vi "Stop Arrival Time TIO.vi"(8 "error in":errorcluster, 10 "Temp File Definition":T1, 11 "Arrival Time Clusters":T2(array[cluster])) -> (0 "error out":errorcluster, 3 "Temp File Definition Out":T1)   [LabVIEW 2009]
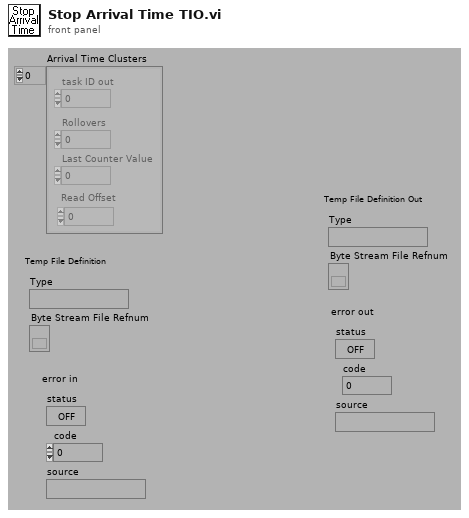
[diagram p1: front panel]
types:
  T1 = cluster{"Type":string, "Byte Stream File Refnum":refnum<file>}
  T2 = cluster{"task ID out":u32, "Rollovers":i32, "Last Counter Value":u32, "Read Offset":i32}[]
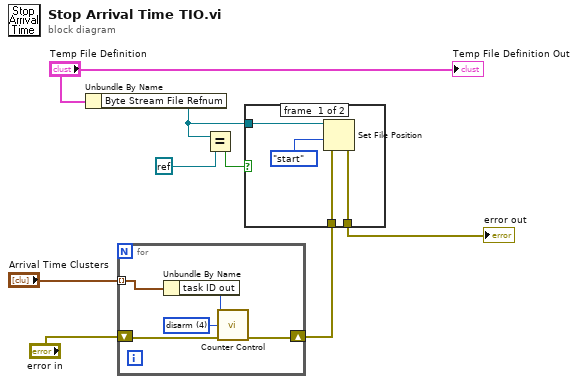
[diagram p0: block diagram]
diagram:
  n1 = Unbundle By Name("Temp File Definition") -> ("Byte Stream File Refnum"=w2:refnum<file>)
  n2 = for {
    tunnel: "Arrival Time Clusters" -> [w12] mode=indexing
    shift-right: [w9] -> w4
    shift-left: "error in" -> [w10]
    w13 = u32 4 items=["program", "reset", "arm", "prepare", "disarm", "count up", "count down", "switch cycle", "snapshot"] ("control code")
    n3 = Unbundle By Name(w12) -> ("task ID out"=w11:u32)
    n4 = call <vilib>:"Counter Control.vi"("task ID"=w11, "control code"=w13, "error in (no error)"=w10) -> ("error out"=w9:errorcluster)  [unwired: 11 in, 1 out]
  }
  n5 = Equal?(x=w2, y=refnum<k0> refnum) -> (x = y?=w7:bool)
  n6 = case shown="False" w7 {
    tunnel: w2 -> [w17 _]
    tunnel: w4 -> [w15 w18]
    tunnel: [w14 w18] -> w3
    frame #0 {
      n7 = Set File Position(refnum=w17, from (0:start)=enum16{"start", "end", "current"}."start" ("pos mode (0:2)"), error in=w15) -> (error out=w14:errorcluster)  [unwired: 1 in, 1 out]
    }
    frame #1 {
    }
  }
  "error out" <- w3
  "Temp File Definition Out" <- "Temp File Definition"
